vi "Shooter Motors.vi"   [LabVIEW 2018]
uses:
  <vilib>/Rock Robotics/WPI/ThirdParty/Phoenix-LabVIEW/Motor Controller/Controls/CTRE_Phoenix_MotorControl_ControlMode.ctl
  <vilib>/Rock Robotics/WPI/ThirdParty/Phoenix-LabVIEW/Motor Controller/Controls/CTRE_Phoenix_MotorControl_NeutralMode.ctl
  Framework/Robot Global Data.vi
types:
  T1 = typedef "CTRE_Phoenix_MotorControl_NeutralMode.ctl" = enum8{"EEPROMSetting", "Override to Coast", "Override to Brake"}
  T2 = typedef "WPI_MotorControlDeviceRef.ctl" = cluster{"DeviceStatus":errorcluster, "Type":T3, "PWM":cluster{"PWM Channel":T4, "DeadBand":T5}, "CAN":cluster{"Device Number":u8, "SetOutput VI Ref":variant, "GetOutput VI Ref":variant, "Enable VI Ref":variant, "Disable VI Ref":variant, "Data":variant}, "Invert":bool, "DIO PWM":cluster{"PWM \"Enable\" Channel":T4, "DIOChannel":T6, "PWM Rate":dbl}}
  T3 = typedef "WPI_MotorControlType.ctl" = enum16{"PWM", "CAN", "DIO PWM"}
  T4 = typedef "FPGA_DIOPWMChannel.ctl" = enum8{"PWM 0", "PWM 1", "PWM 2", "PWM 3", "PWM 4", "PWM 5", "PWM 6", "PWM 7", "PWM 8", "PWM 9", "PWM MXP 0", "PWM MXP 1", "PWM MXP 2", "PWM MXP 3", "PWM MXP 4", "PWM MXP 5", "PWM MXP 6", "PWM MXP 7", "PWM MXP 8", "PWM MXP 9", "Invalid"}
  T5 = typedef "WPI_PWMDeadband.ctl" = cluster{"Name":string, "maxPositivePwm":i32, "minPositivePwm":i32, "centerPwm":i32, "maxNegativePwm":i32, "minNegativePwm":i32, "angularRange":u16}
  T6 = typedef "FPGA_DIOChannel.ctl" = enum8{"DIO 0", "DIO 1", "DIO 2", "DIO 3", "DIO 4", "DIO 5", "DIO 6", "DIO 7", "DIO 8", "DIO 9", "DIO MXP 0", "DIO MXP 1", "DIO MXP 2", "DIO MXP 3", "DIO MXP 4", "DIO MXP 5", "DIO MXP 6", "DIO MXP 7", "DIO MXP 8", "DIO MXP 9", "DIO MXP 10", "DIO MXP 11", "DIO MXP 12", "DIO MXP 13", "DIO MXP 14", "DIO MXP 15", "SPI Port CS1", "SPI Port CS2", "SPI Port CS3", "SPI Port MISO", "SPI Port MOSI", "Invalid"}
  T7 = typedef "CTRE_Phoenix_MotorControl_ControlMode.ctl" = u16
  T8 = typedef "WPI_DriverStationRobotMode2.ctl" = enum16{"Autonomous Disabled", "Autonomous Enabled", "Teleop Disabled", "Teleop Enabled", "Disconnected", "Finish", "Test Disabled", "Test Enabled", "Emergency Stopped"}
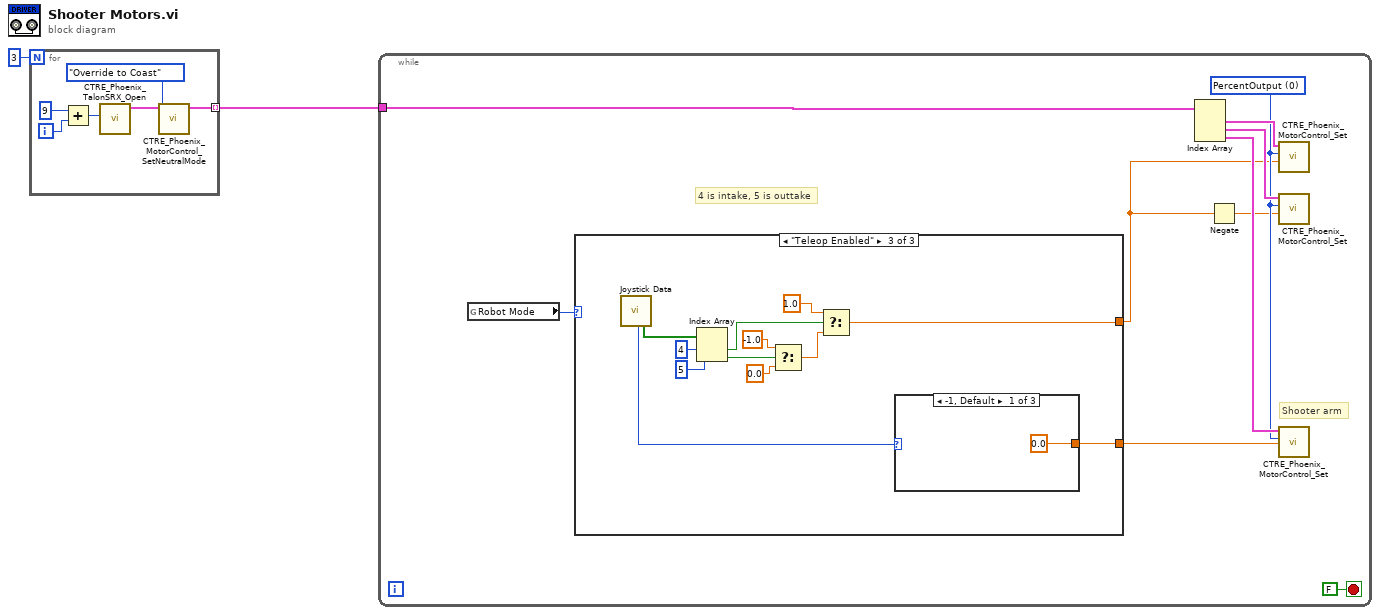
[diagram p0: block diagram]
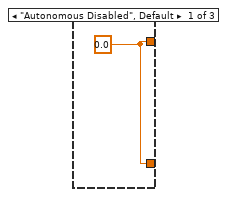
[diagram p2: hidden frame]
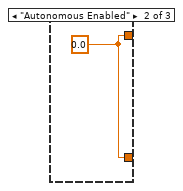
[diagram p3: hidden frame]
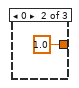
[diagram p4: hidden frame]
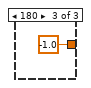
[diagram p5: hidden frame]
diagram:
  n1 = for {
    N: 3 -> [_]
    tunnel: [w3] -> w1 mode=indexing
    i -> [w6]
    n2 = Add(x=9, y=w6) -> (x+y=w4:i32)
    n3 = call <vilib>:"CTRE_Phoenix_TalonSRX_Open.vi"("Device Number"=w4) -> ("CAN Talon SRX Ref"=w8:T2)  [unwired: 9 in, 1 out]
    n4 = call <vilib>:"CTRE_Phoenix_MotorControl_SetNeutralMode.vi"("Motor Control Neutral Mode"=CTRE_Phoenix_MotorControl_NeutralMode."Override to Coast", "PhoenixMotorControlDevRef"=w8) -> ("PhoenixMotorControlDevRef"=w3:T2)  [unwired: 8 in, 1 out]
  }
  n5 = while {
    tunnel: w1 -> [w17]
    stop <- FALSE stop-if-true
    w12 = T7 0 items=["PercentOutput"=0, "Position"=1, "Velocity"=2, "Current"=3, "Follower"=5, "MotionProfile"=6, "MotionMagic"=7, "MotionProfileArc"=10, "Disabled"=15] ("Control Mode")
    # "4 is intake, 5 is outtake"
    # "Shooter arm"
    n6 = global read "Robot Global Data.vi" "Robot Mode"() -> (w13:T8)
    n7 = case shown="\"Teleop Enabled\"" w13 {
      tunnel: [w19 w20 w31] -> w11
      tunnel: [w19 w20 w21] -> w9
      frame "Autonomous Disabled", Default {
        w19 = 0.0
      }
      frame "Autonomous Enabled" {
        w20 = 0.0
      }
      frame "Teleop Enabled" {
        n8 = call "Joystick Data.vi"() -> ("Controller POV Out"=w32:i16, "Controller Buttons Out"=w30:bool[])  [unwired: 12 in, 6 out]
        n9 = Index Array(array=w30, index #1=4 ("index"), index #2=5 ("index")) -> (element #1=w27:bool, element #2=w25:bool)
        n10 = Select(t=-1.0, s=w25, f=0.0) -> (s? t:f=w23:dbl)
        n11 = Select(t=1.0, s=w27, f=w23) -> (s? t:f=w21:dbl)
        n12 = case shown="-1, Default" w32 {
          tunnel: [0.0 ("Output") 1.0 ("Output") -1.0 ("Output")] -> w31
          frame -1, Default {
          }
          frame 0 {
          }
          frame 180 {
          }
        }
      }
    }
    n13 = Index Array(array=w17) -> (element #1=w16:T2, element #2=w15:T2, element #3=w14:T2)  [unwired: 3 in]
    n14 = Negate(x=w9) -> (-x=w10:dbl)
    n15 = call <vilib>:"CTRE_Phoenix_MotorControl_Set.vi"("Output"=w9, "Control Mode"=w12, "PhoenixMotorControlDevRef"=w16) -> ()  [unwired: 7 in, 2 out]
    n16 = call <vilib>:"CTRE_Phoenix_MotorControl_Set.vi"("Output"=w10, "Control Mode"=w12, "PhoenixMotorControlDevRef"=w15) -> ()  [unwired: 7 in, 2 out]
    n17 = call <vilib>:"CTRE_Phoenix_MotorControl_Set.vi"("Output"=w11, "Control Mode"=w12, "PhoenixMotorControlDevRef"=w14) -> ()  [unwired: 7 in, 2 out]
  }
